vi "list all targets.vi"() -> (3 "all targets":T1[](array[typedef]))   [LabVIEW 2013, in "TBM configuration.lvclass"]
doc: "A helper function which provides a list of all target types supported in the framework."
uses:
  TBM configuration.lvclass
  Target Types.ctl
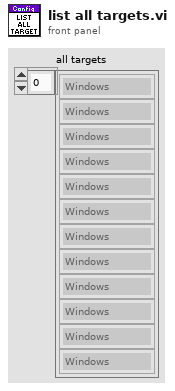
[diagram p1: front panel]
types:
  T1 = typedef "TBM configuration.lvclass/Target Types.ctl" = enum16{"Windows", "Mac", "Linux", "Linux RT", "VxWorks", "Pharlap", "Other"}
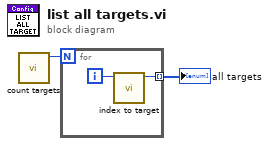
[diagram p0: block diagram]
diagram:
  n1 = call "count targets.vi"() -> ("target type count"=w2:i32)  [unwired: 11 in]
  n2 = for {
    N: w2 -> [_]
    tunnel: [w3] -> w1 mode=indexing
    i -> [w4]
    n3 = call "index to target.vi"("i32"=w4) -> ("target"=w3:T1)  [unwired: 10 in]
  }
  "all targets" <- w1
